vi "Main.vi"(8 "error in (no error)":errorcluster, 11 "AutofocusBase in":refnum<class "Autofocus.lvclass">) -> (0 "error out":errorcluster, 3 "component":refnum<class "Autofocus.lvclass">)   [LabVIEW 2012, in "Autofocus.lvclass"]
doc: "Main VI of the component."
uses:
  Autofocus.lvclass
  <vilib>/Distrio/Murmex/Murmex/Murmex.lvclass
  <vilib>/Distrio/Murmex/InitialiseMessage/InitialiseMessage.lvclass
  <vilib>/Distrio/Murmex/TerminateMessage/TerminateMessage.lvclass
  <vilib>/Distrio/Murmex/StopMessage/StopMessage.lvclass
  <vilib>/Distrio/Murmex/ConfigureMessage/ConfigureMessage.lvclass
  <vilib>/Distrio/Murmex/Message/Message.lvclass
  <vilib>/Distrio/Murmex/Murmex/update_cluster.ctl
  <vilib>/Distrio/Murmex/Murmex/command_enum.ctl
  ROI size.ctl
  Sharpness Measure.ctl
  Search algorithm.ctl
  image acquisition mode.ctl
panel:
  in  "button::configure":bool
  out "terminate?":bool=TRUE
  in  "button::stop":bool
  in  "button::quit":bool
  in  "Tab Control":T1(tab)
  in  "Image acquisition mode":T2
  in  "Frames in focus stack":u16
  in  "focus stage stop position":dbl[unit] caption="stop position"
  in  "focus stage start position":dbl[unit] caption="start position"
  out "progress bar tomo":dbl(slide) caption="progress bar" scale=0.0..100.0
  out "progress bar stack":dbl(slide) caption="progress bar" scale=0.0..100.0
  in  "HC step size":dbl[unit]
  out "z2":dbl[unit]
  out "z1":dbl[unit]
  out "y":dbl[unit]
  out "x":dbl[unit]
  in  "number of checkpoints":u16 max=50 step=1
  in  "brightest pecentage":dbl
  in  "intensity threshold":dbl
  out "Latest Focus curve":cluster{"x array":dbl[], "y array":dbl[]}(graph)
  in  "Search Algorithm":T3
  in  "Sharpness measure":T4
  out "current_position_focus":dbl[unit] caption="focus stage current position"
  out "Linear fit through stack":cluster{"x array":dbl[], "y array":dbl[]}(graph)
  in  "Region sampling":bool
  in  "ROI size":T5 items=["50x50"=50, "100x100"=100, "250x250"=250]
  in  "button::send":bool
  in  "ID":string="stage"
  in  "command":T6
  in  "Generic command":string
  out "log":string
  # "Stacks"
  # "Checkpoints"
  # "Focus stage search range"
  # "Measure and Search"
  # "current stack"
  # "Images"
  # "Tomo"
  # "Region sampling"
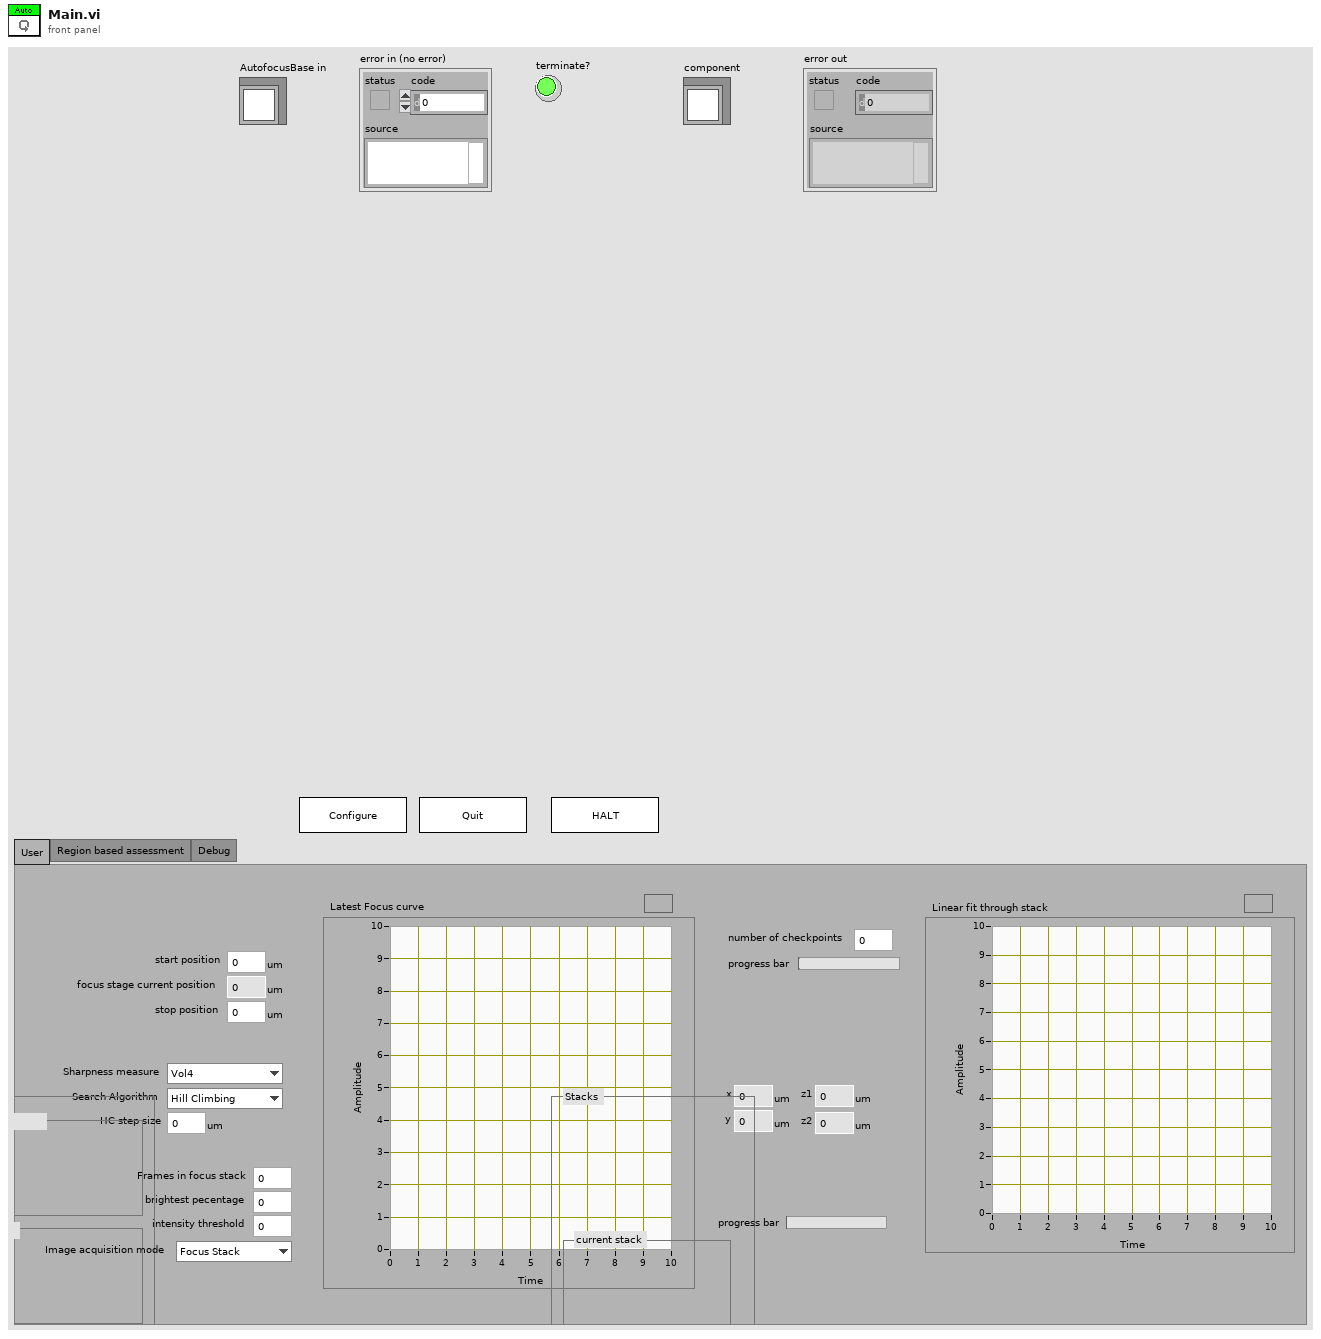
[diagram p1: front panel]
types:
  T1 = enum32{"User", "Region based assessment", "Debug"}
  T2 = typedef "Autofocus.lvclass/image acquisition mode.ctl" = enum16{"Focus Stack", "Single Frame"}
  T3 = typedef "Autofocus.lvclass/Search algorithm.ctl" = enum16{"Hill Climbing", "HC+GS"}
  T4 = typedef "Autofocus.lvclass/Sharpness Measure.ctl" = enum16{"Vol4", "Gradient Square"}
  T5 = typedef "Autofocus.lvclass/ROI size.ctl" = u16
  T6 = typedef "Murmex.lvlib/Murmex.lvclass/command_enum.ctl" = enum16{"null", "initialise", "reset", "terminate", "acknowledge", "update", "inspect", "inform", "proceed", "start", "stop", "fetch", "configure", "generic"}
  T7 = enum8{"Enabled", "Disabled", "Disabled and Grayed Out"}
  T8 = typedef "Murmex.lvlib/Murmex.lvclass/update_cluster.ctl" = cluster{"target ID":string, "key chains":string[], "values":variant[]}
  T9 = typedef "Murmex.lvlib/Murmex.lvclass/Event type enumerations.ctl" = enum16{"before", "after"}
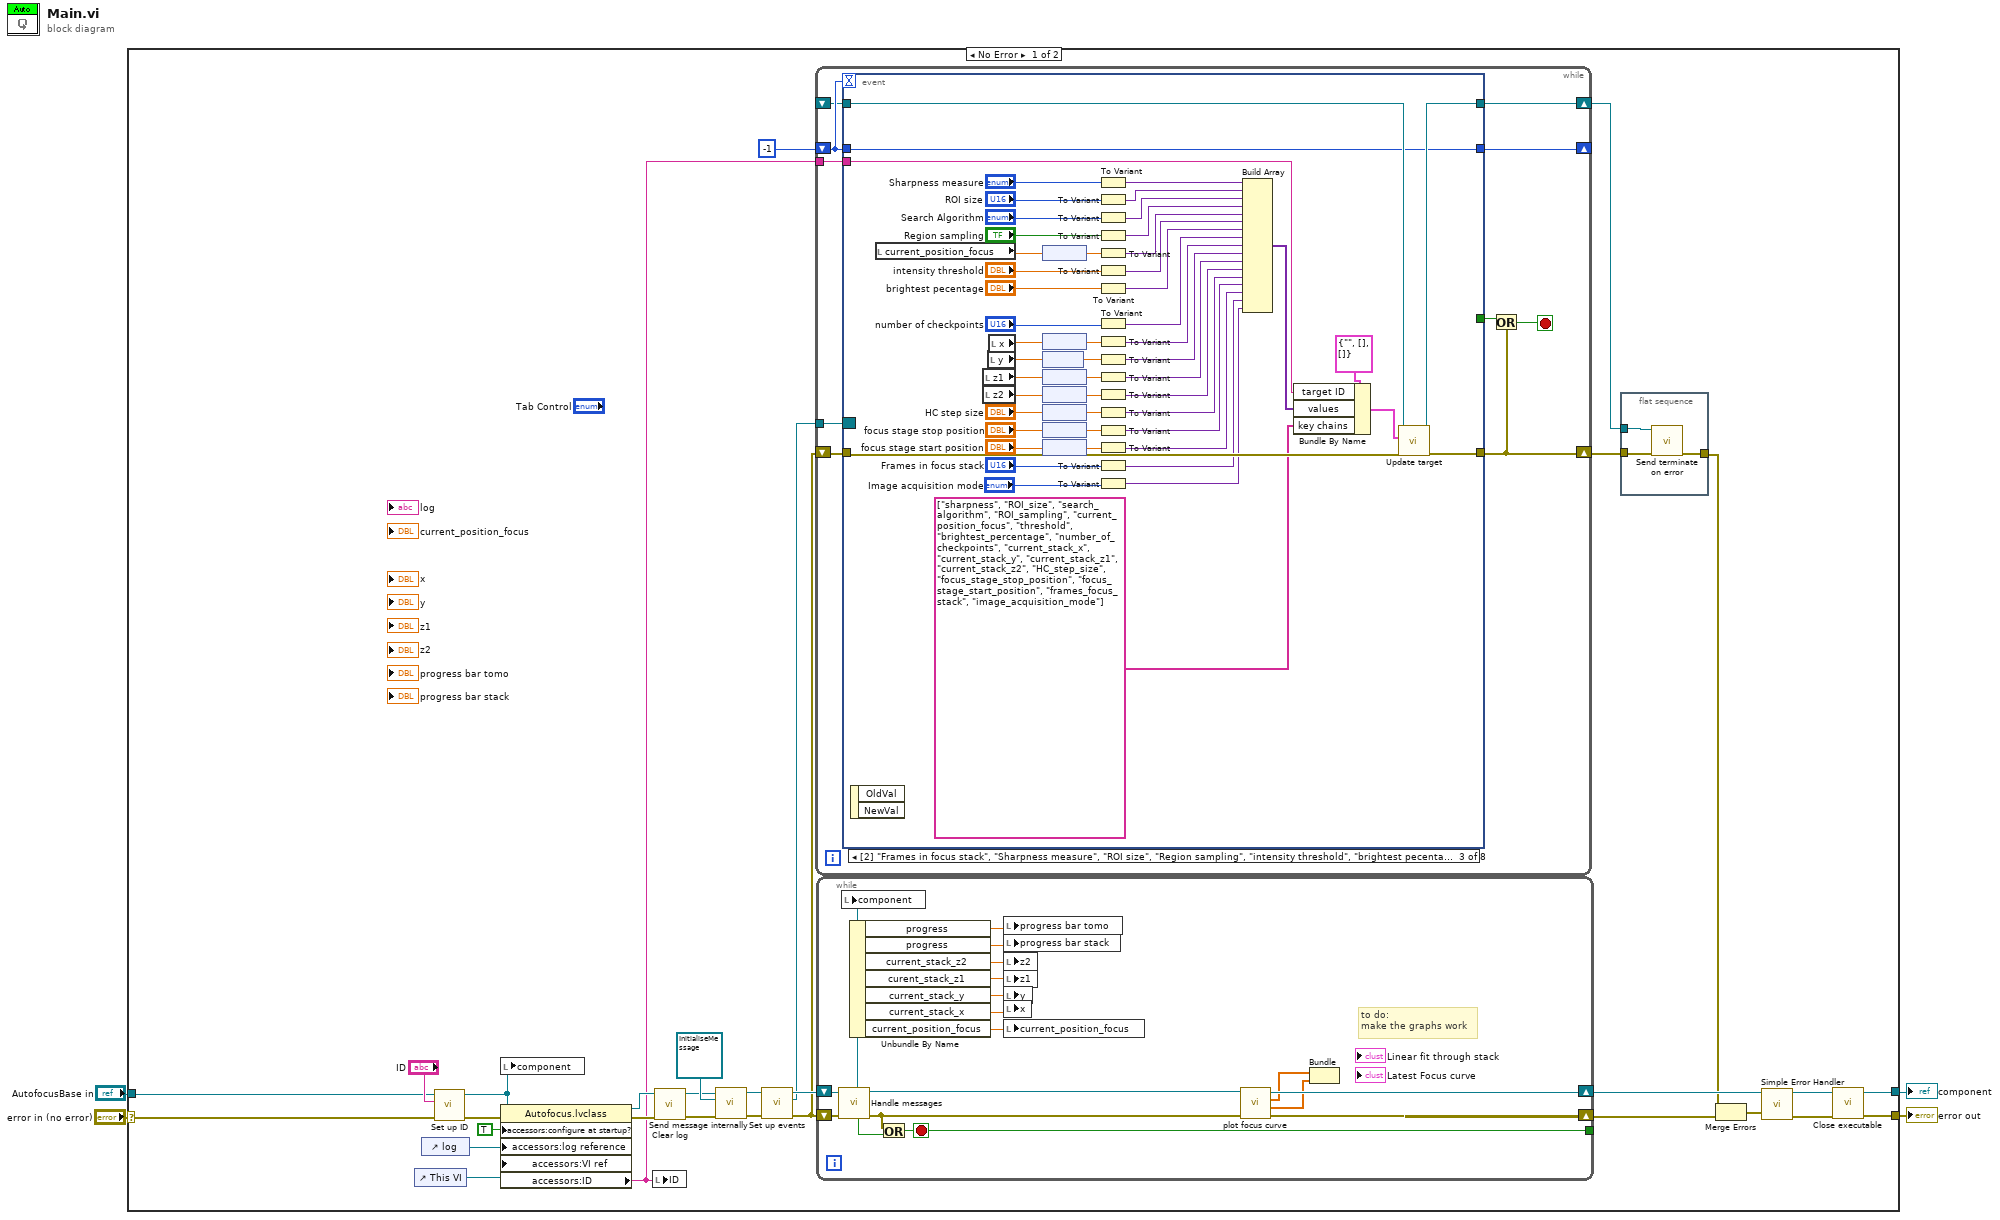
[diagram p0: block diagram]
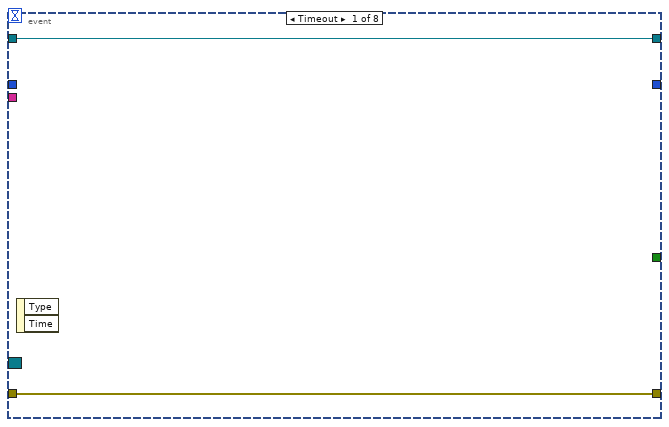
[diagram p2: hidden frame]
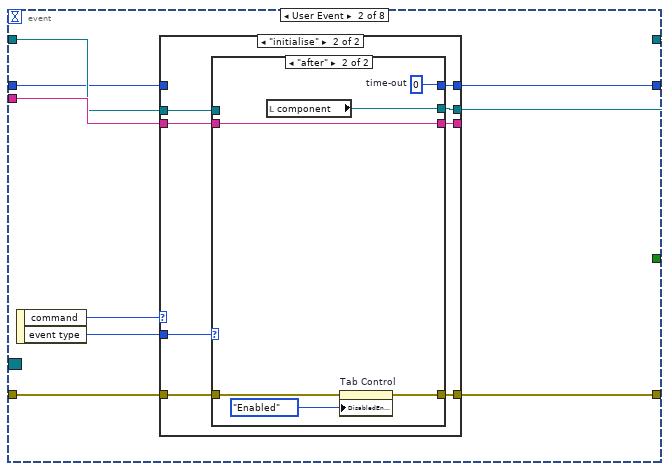
[diagram p3: hidden frame]
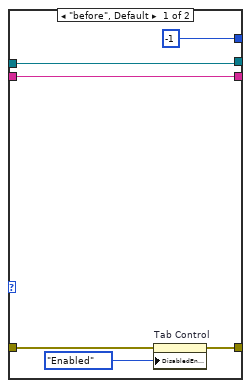
[diagram p5: hidden frame]
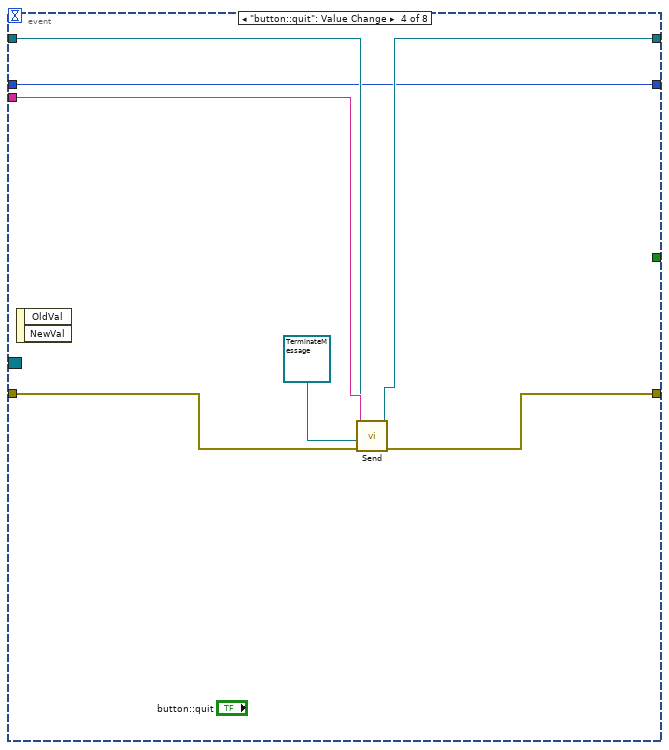
[diagram p6: hidden frame]
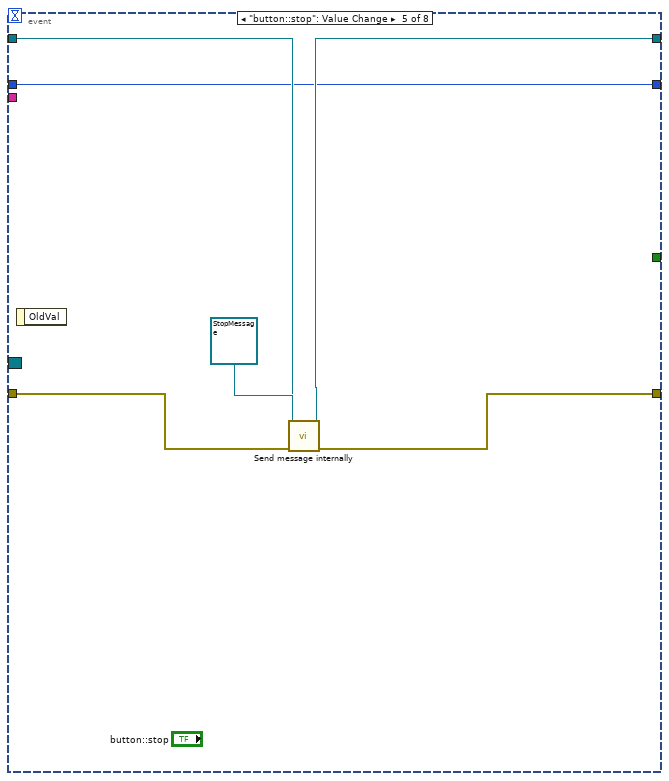
[diagram p7: hidden frame]
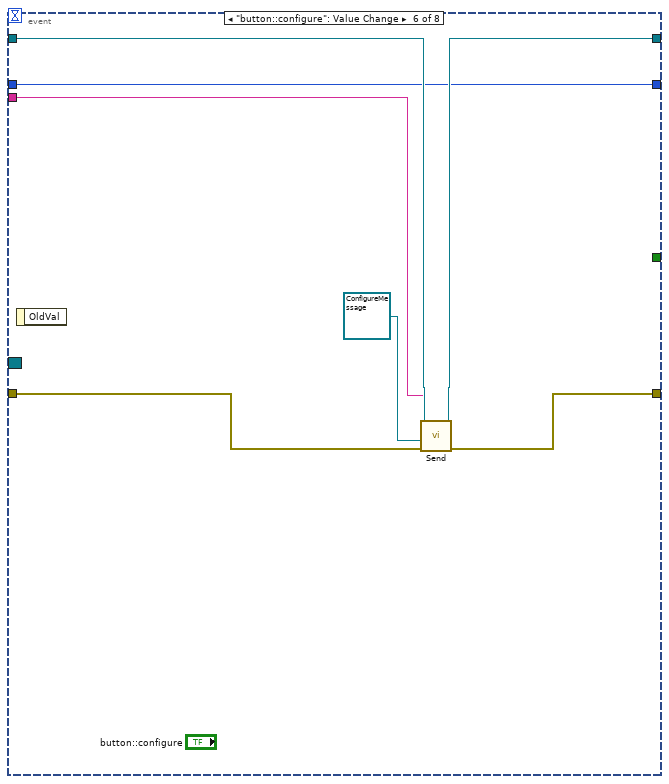
[diagram p8: hidden frame]
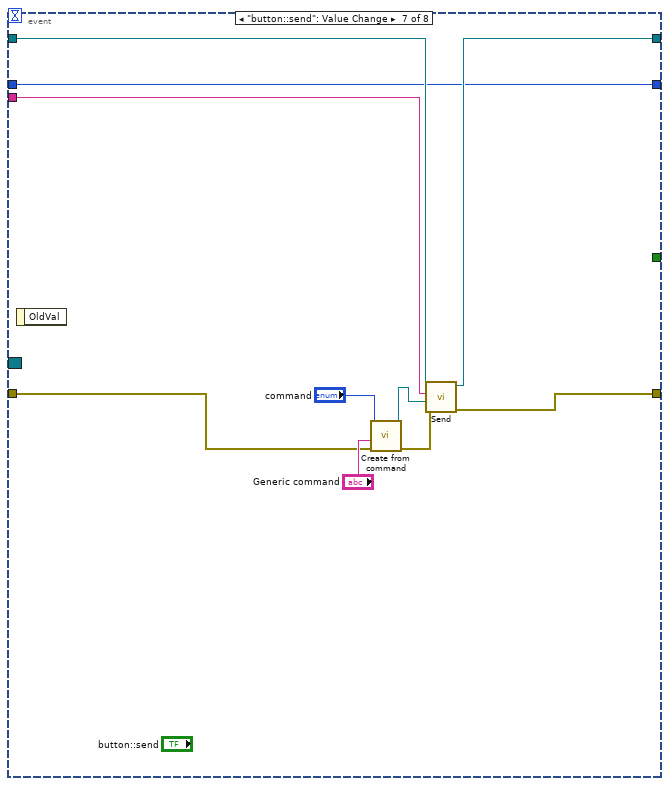
[diagram p9: hidden frame]
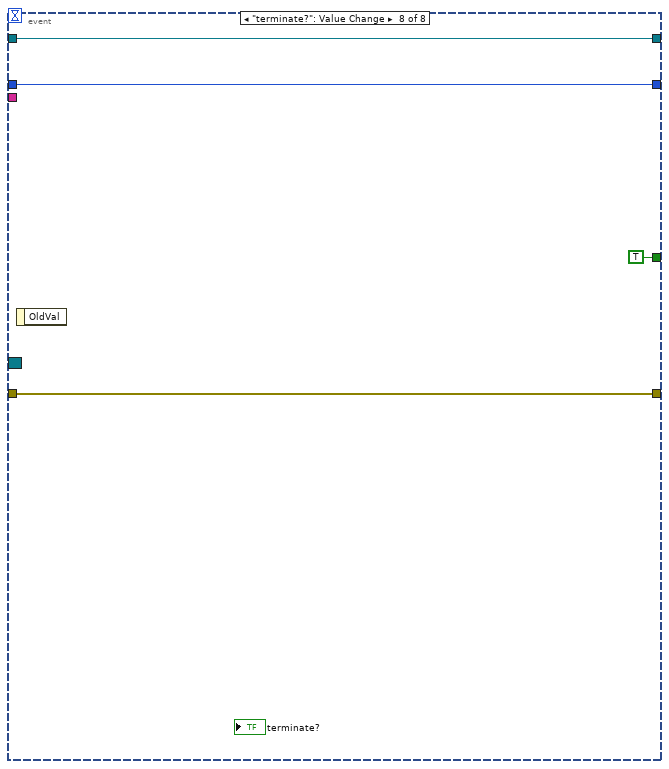
[diagram p10: hidden frame]
diagram:
  n1 = case shown="No Error" "error in (no error)" {
    selector: "error in (no error)" -> [w31 w186]
    tunnel: "AutofocusBase in" -> [w32 w185]
    tunnel: [w9 w186] -> w2
    tunnel: [w8 w185] -> w1
    frame No Error {
      n2 = control-ref of="This VI"() -> (w28:refnum<vi>)
      n3 = control-ref of="log"() -> (w10:refnum<vi>)
      n4 = call <vilib>:"Set up ID.vi"("error in (no error)"=w31, "component ID"="ID", "MurmexBase in"=w32) -> ("error out"=w30:errorcluster, "MurmexBase out"=w20:refnum<class "Autofocus.lvclass">)  [unwired: 6 in, 1 out]
      n5 = local write "component"(w20) -> ()
      n6 = property class="Autofocus.lvclass"(reference=w20, error in=w30, "accessors:configure at startup?"=TRUE ("configure at startup?"), "accessors:log reference"=w10, "accessors:VI ref"=w28) -> (reference out=w21:refnum<class "Autofocus.lvclass">, error out=w22:errorcluster, "accessors:ID"=w11:string)
      n7 = local write "ID"(w11) -> ()
      n8 = call <vilib>:"Clear log.vi"("error in (no error)"=w22, "MurmexBase in"=w21) -> ("error out"=w23:errorcluster, "MurmexBase out"=w24:refnum<class "Autofocus.lvclass">)  [unwired: 8 in]
      n9 = call <vilib>:"Send message internally.vi"("error in (no error)"=w23, "Message"=refnum<class "InitialiseMessage.lvclass"> refnum ("Distrio Murmex 1.1:InitialiseMessage"), "Murmex in"=w24) -> ("error out"=w26:errorcluster, "Murmex out"=w27:refnum<class "Autofocus.lvclass">)  [unwired: 7 in]
      n10 = call <vilib>:"Set up events.vi"("error in (no error)"=w26, "MurmexBase in"=w27) -> ("error out"=w13:errorcluster, "Event Registration Refnum"=w14:refnum<event-registration>, "MurmexBase out"=w19:refnum<class "Autofocus.lvclass">)  [unwired: 7 in]
      n11 = while {
        tunnel: w14 -> [w46]
        shift-right: [w38] -> w6
        shift-left: w13 -> [w45]
        shift-right: [w40] -> _
        shift-left: -1 -> [w44]
        tunnel: w11 -> [w43]
        shift-right: [w42] -> w7
        shift-left: _ -> [w41]
        stop <- w37 stop-if-true
        n12 = event shown="[2] \"Frames in focus stack\", \"Sharpness measure\", \"ROI size\", \"Region sampling\", \"intensity threshold\", \"brightest pecentage\", \"number of checkpoints\", \"focus stage stop position\", \"focus stage start position\", \"HC step size\", \"Search Algorithm\", \"Image acquisition mode\": Value Change" {
          selector: w46 -> [_ _ _ _ _ _ _ _]
          dyn-events: _ -> [_ _ _ _ _ _ _ _]
          timeout: w44 -> [_ _ _ _ _ _ _ _]
          tunnel: w45 -> [w48 w57 w127 w139 w145 w152 w159 w167]
          tunnel: w44 -> [_ w49 w87 w134 w141 w147 w154 w164]
          tunnel: w43 -> [_ w56 w124 w137 _ w148 w155 _]
          tunnel: [w47 w53 w122 w135 w142 w149 w156 w165] -> w42
          tunnel: w41 -> [w47 w52 w123 w136 w143 w150 w157 w165]
          tunnel: [_ w51 w87 w134 w141 w147 w154 w164] -> w40
          tunnel: [w48 w50 w126 w138 w144 w151 w158 w167] -> w38
          tunnel: [_ _ _ _ _ _ _ TRUE] -> w39
          event Timeout {
            n13 = event-data() -> ()  [unwired: 1 in, 2 out]
          }
          event User Event {
            n14 = event-data() -> ("command"=w55:T6, "event type"=w54:T9)  [unwired: 1 in]
            n15 = case shown="\"initialise\"" w55 {
              tunnel: w57 -> [w60 w69]
              tunnel: [w60 w68] -> w50
              tunnel: w56 -> [w61 w67]
              tunnel: [w58 w66] -> w53
              tunnel: [w61 w65] -> _
              tunnel: w54 -> [_ w64]
              tunnel: [w59 w63] -> w51
              tunnel: w52 -> [w58 w62]
              tunnel: w49 -> [w59 _]
              frame "null", Default {
              }
              frame "initialise" {
                n16 = case shown="\"after\"" w64 {
                  tunnel: [w74 w80] -> w68
                  tunnel: w69 -> [w75 w81]
                  tunnel: w67 -> [w72 w77]
                  tunnel: [w70 w79] -> w66
                  tunnel: [w72 w77] -> w65
                  tunnel: [-1 w76] -> w63
                  tunnel: w62 -> [w70 _]
                  frame "before", Default {
                    n17 = property on="Tab Control" class="TabCtl (strict)"(error in=w75, "DisabledEnum"=T7."Enabled" ("Disabled")) -> (error out=w74:errorcluster)  [unwired: 1 in, 1 out]
                  }
                  frame "after" {
                    w76 = 0  # time-out
                    n18 = local read "component"() -> (w79:refnum<class "Autofocus.lvclass">)
                    n19 = property on="Tab Control" class="TabCtl (strict)"(error in=w81, "DisabledEnum"=T7."Enabled" ("Disabled")) -> (error out=w80:errorcluster)  [unwired: 1 in, 1 out]
                  }
                }
              }
            }
          }
          event "Frames in focus stack", "Region sampling", "intensity threshold", "brightest pecentage", "number of checkpoints", "focus stage stop position", "focus stage start position", "HC step size": Value Change {
            n20 = event-data() -> ()  [unwired: 1 in, 2 out]
            n21 = local read "current_position_focus"() -> (w114:dbl[unit])
            n22 = local read "z1"() -> (w106:dbl[unit])
            n23 = local read "z2"() -> (w105:dbl[unit])
            n24 = local read "y"() -> (w100:dbl[unit])
            n25 = local read "x"() -> (w107:dbl[unit])
            n26 = node(w114) -> (w96:dbl)
            n27 = node(w107) -> (w101:dbl)
            n28 = node(w100) -> (w99:dbl)
            n29 = node(w106) -> (w98:dbl)
            n30 = node(w105) -> (w97:dbl)
            n31 = node("HC step size") -> (w94:dbl)
            n32 = node("focus stage stop position") -> (w90:dbl)
            n33 = node("focus stage start position") -> (w86:dbl)
            n34 = To Variant(anything="Sharpness measure") -> (Variant=w131:variant)
            n35 = To Variant(anything="ROI size") -> (Variant=w130:variant)
            n36 = To Variant(anything="Search Algorithm") -> (Variant=w129:variant)
            n37 = To Variant(anything="Region sampling") -> (Variant=w125:variant)
            n38 = To Variant(anything=w96) -> (Variant=w113:variant)
            n39 = To Variant(anything="intensity threshold") -> (Variant=w112:variant)
            n40 = To Variant(anything="brightest pecentage") -> (Variant=w111:variant)
            n41 = To Variant(anything="number of checkpoints") -> (Variant=w110:variant)
            n42 = To Variant(anything=w101) -> (Variant=w108:variant)
            n43 = To Variant(anything=w99) -> (Variant=w104:variant)
            n44 = To Variant(anything=w98) -> (Variant=w103:variant)
            n45 = To Variant(anything=w97) -> (Variant=w102:variant)
            n46 = To Variant(anything=w94) -> (Variant=w93:variant)
            n47 = To Variant(anything=w90) -> (Variant=w89:variant)
            n48 = To Variant(anything=w86) -> (Variant=w88:variant)
            n49 = To Variant(anything="Frames in focus stack") -> (Variant=w84:variant)
            n50 = To Variant(anything="Image acquisition mode") -> (Variant=w82:variant)
            n51 = Build Array(w131, w130, w129, w125, w113, w112, w111, w110, w108, w104, w103, w102, w93, w89, w88, w84, w82) -> (w128:variant[])
            n52 = Bundle By Name(cluster=T8 {"target ID"="", "key chains"=[], "values"=[]} ("update cluster"), "target ID"=w124, "values"=w128, "key chains"=string[] ["sharpness", "ROI_size", "search_algorithm", "ROI_sampling", "current_position_focus", "threshold", "brightest_percentage", "number_of_checkpoints", "current_stack_x", "current_stack_y", "current_stack_z1", "current_stack_z2", "HC_step_size", "focus_stage_stop_position", "focus_stage_start_position", "frames_focus_stack", "image_acquisition_mode"]) -> (w133:T8)
            n53 = call <vilib>:"Update target.vi"("error in (no error)"=w127, "update cluster"=w133, "MurmexBase in"=w123) -> ("error out"=w126:errorcluster, "MurmexBase out"=w122:refnum<class "Autofocus.lvclass">)  [unwired: 7 in]
          }
          event "button::quit": Value Change {
            n54 = event-data() -> ()  [unwired: 1 in, 2 out]
            n55 = call <vilib>:"Send.vi"("error in (no error)"=w139, "Message"=refnum<class "TerminateMessage.lvclass"> refnum ("Murmex.lvlib:TerminateMessage"), "recipient"=w137, "Murmex in"=w136) -> ("error out"=w138:errorcluster, "Murmex out"=w135:refnum<class "Autofocus.lvclass">)  [unwired: 6 in]
          }
          event "button::stop": Value Change {
            n56 = event-data() -> ()  [unwired: 1 in, 1 out]
            n57 = call <vilib>:"Send message internally.vi"("error in (no error)"=w145, "Message"=refnum<class "StopMessage.lvclass"> refnum ("Distrio Murmex 1.5:StopMessage"), "Murmex in"=w143) -> ("error out"=w144:errorcluster, "Murmex out"=w142:refnum<class "Autofocus.lvclass">)  [unwired: 7 in]
          }
          event "button::configure": Value Change {
            n58 = event-data() -> ()  [unwired: 1 in, 1 out]
            n59 = call <vilib>:"Send.vi"("error in (no error)"=w152, "Message"=refnum<class "ConfigureMessage.lvclass"> refnum ("Distrio Murmex 1.1:ConfigureMessage"), "recipient"=w148, "Murmex in"=w150) -> ("error out"=w151:errorcluster, "Murmex out"=w149:refnum<class "Autofocus.lvclass">)  [unwired: 6 in]
          }
          event "button::send": Value Change {
            n60 = event-data() -> ()  [unwired: 1 in, 1 out]
            n61 = call <vilib>:"Create from command.vi"("error in (no error)"=w159, "generic command"="Generic command", "command"="command") -> ("error out"=w162:errorcluster, "Message out"=w161:refnum<class "Message.lvclass">)  [unwired: 7 in]
            n62 = call <vilib>:"Send.vi"("error in (no error)"=w162, "Message"=w161, "recipient"=w155, "Murmex in"=w157) -> ("error out"=w158:errorcluster, "Murmex out"=w156:refnum<class "Autofocus.lvclass">)  [unwired: 6 in]
          }
          event "terminate?": Value Change {
            n63 = event-data() -> ()  [unwired: 1 in, 1 out]
          }
        }
        n64 = Or(x=w39, y=w38) -> (x .or. y?=w37:bool)
      }
      n65 = while {
        shift-right: [w180] -> w15
        shift-left: w19 -> [w183]
        shift-right: [w178] -> w16
        shift-left: w13 -> [w184]
        tunnel: [w181] -> _
        stop <- w181 stop-if-true
        # "to do:\nmake the graphs work"
        n66 = call <vilib>:"Handle messages.vi"("error in (no error)"=w184, "Murmex in"=w183) -> ("error out"=w179:errorcluster, "Murmex out"=w175:refnum<class "Autofocus.lvclass">, "terminated?"=w182:bool)  [unwired: 7 in]
        n67 = local write "component"(w175) -> ()
        n68 = Unbundle By Name(w175) -> ("progress"=w168:dbl, "progress"=w169:dbl, "current_stack_z2"=w170:dbl[unit], "curent_stack_z1"=w171:dbl[unit], "current_stack_y"=w172:dbl[unit], "current_stack_x"=w173:dbl[unit], "current_position_focus"=w174:dbl[unit])
        n69 = Or(x=w179, y=w182) -> (x .or. y?=w181:bool)
        n70 = local write "progress bar tomo"(w168) -> ()
        n71 = local write "progress bar stack"(w169) -> ()
        n72 = local write "z2"(w170) -> ()
        n73 = local write "z1"(w171) -> ()
        n74 = local write "y"(w172) -> ()
        n75 = local write "x"(w173) -> ()
        n76 = local write "current_position_focus"(w174) -> ()
        n77 = call-dynamic "plot focus curve.vi"("error in (no error)"=w179, "Autofocus in"=w175) -> ("error out"=w178:errorcluster, "x array"=w176:dbl[], "y array"=w177:dbl[], "Autofocus out"=w180:refnum<class "Autofocus.lvclass">)  [unwired: 6 in]
        n78 = Bundle("y array"=w177, "x array"=w176) -> ()  [unwired: 1 in, 1 out]
      }
      n79 = flat-sequence {
        tunnel: w6 -> [w36]
        tunnel: [w35] -> w5
        tunnel: w7 -> [w34]
        frame #0 {
          n80 = call <vilib>:"Send terminate on error.vi"("error in (no error)"=w36, "Murmex in"=w34) -> ("error out"=w35:errorcluster)  [unwired: 8 in, 1 out]
        }
      }
      n81 = Merge Errors(w5, w16) -> (w17:errorcluster)
      n82 = call <vilib>:"Simple Error Handler.vi"("error in (no error)"=w17) -> ("error out"=w18:errorcluster)  [unwired: 4 in, 4 out]
      n83 = call <vilib>:"Close executable.vi"("error in (no error)"=w18, "MurmexBase in"=w15) -> ("error out"=w9:errorcluster, "MurmexBase out"=w8:refnum<class "Autofocus.lvclass">)  [unwired: 8 in]
    }
    frame Error {
    }
  }
  "error out" <- w2
  "component" <- w1
